vi "Launcher.vi"() -> ()   [LabVIEW 2020]
uses:
  UI Actor/UI Actor.lvclass
  C:/Program Files (x86)/National Instruments/LabVIEW 2020/vi.lib/ActorFramework/Actor/Actor.lvclass
  UI Actor/UI Actor.lvclass/UI Actor.ctl
  UI Actor/Set Coins.vi
  UI Actor/Set Products.vi
  UI Actor/Set Language.vi
  <vilib>/ActorFramework/Actor/Actor.lvclass
panel:
  in  "Language":enum16{"ESP", "ENG"}(ring)
  in  "Products":enum16{"Coca", "Sabritas"}(ring)
  in  "Coins":enum16{"MXN", "USD"}(ring)
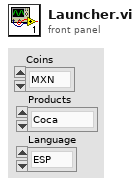
[diagram p1: front panel]
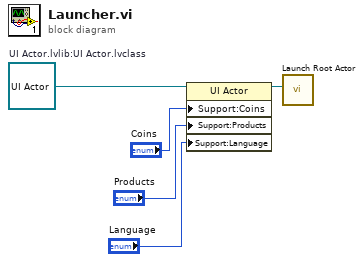
[diagram p0: block diagram]
diagram:
  w5 = refnum<class "UI Actor.lvclass"> refnum  # UI Actor.lvlib:UI Actor.lvclass
  n1 = property class="UI Actor"(reference=w5, "Support:Coins"="Coins", "Support:Products"="Products", "Support:Language"="Language") -> (reference out=w4:refnum<class "UI Actor.lvclass">)  [unwired: 1 in, 1 out]
  n2 = call <vilib>:"Launch Root Actor.vi"("Actor"=w4) -> ()  [unwired: 9 in, 2 out]
